vi "main.vi"() -> ()   [LabVIEW 2019]
uses:
  Controls/States.ctl
  Controls/Data.ctl
panel:
  in  "Exit":bool
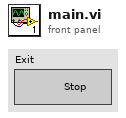
[diagram p1: front panel]
types:
  T1 = typedef "Data.ctl" = cluster{"Data":dbl[], "Info":string}
  T2 = typedef "States.ctl" = enum16{"Inizialize", "Wait for event", "Calculate", "Clear", "Exit"}
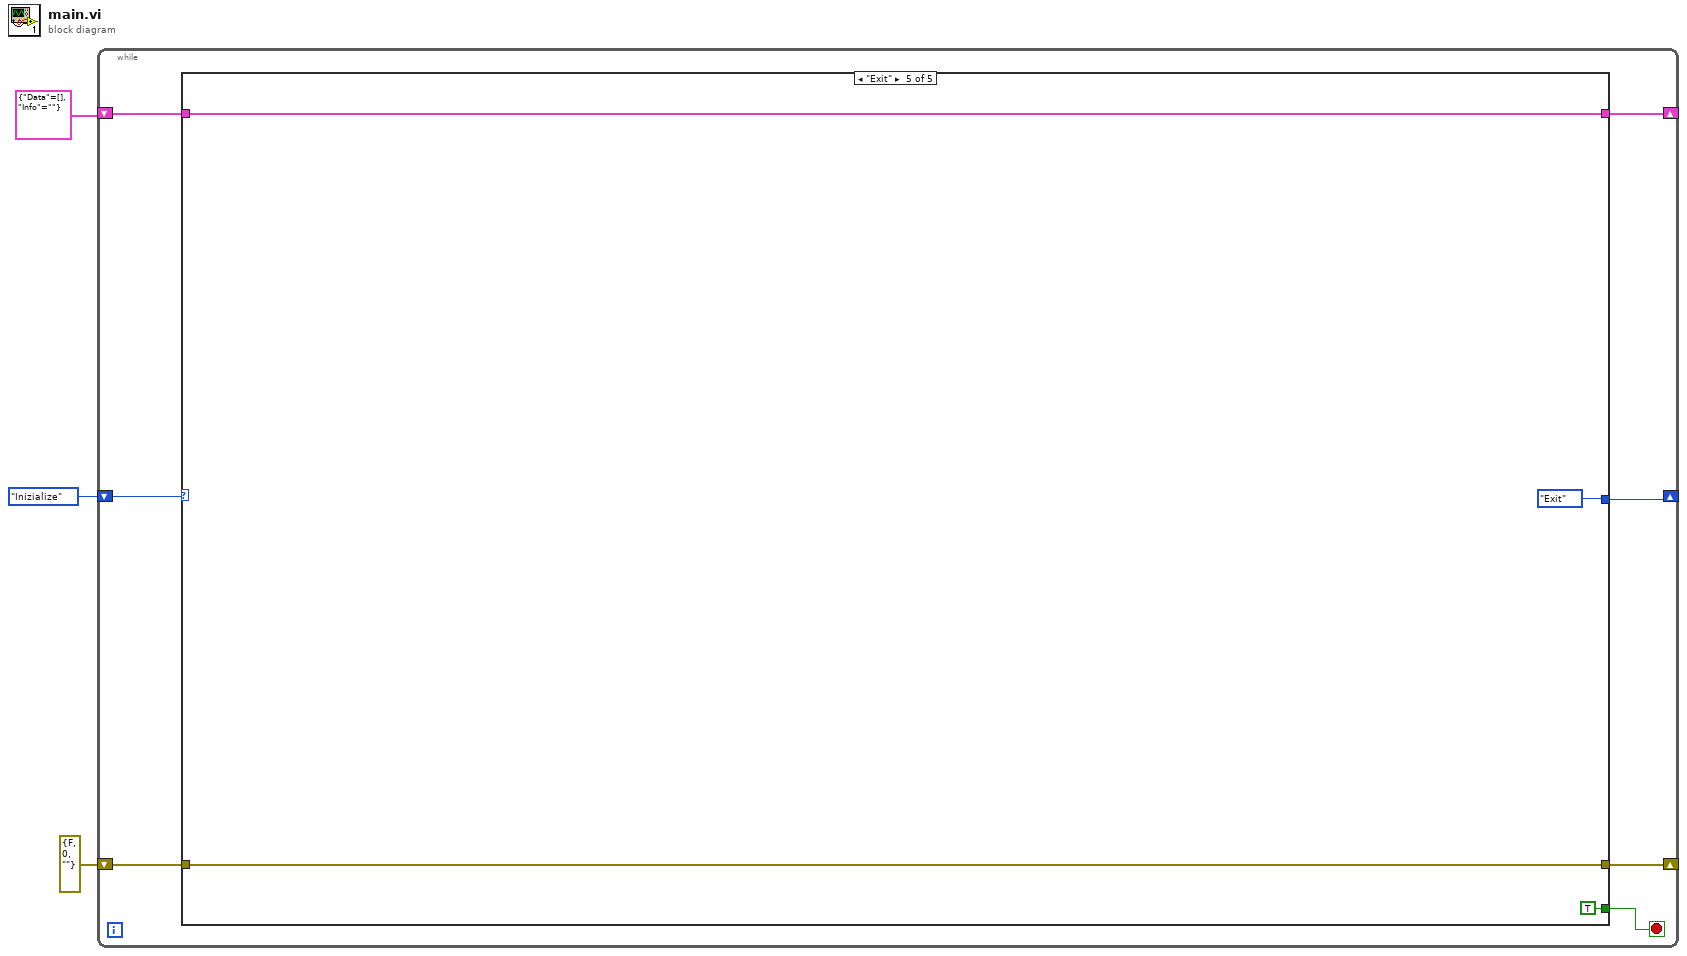
[diagram p0: block diagram]
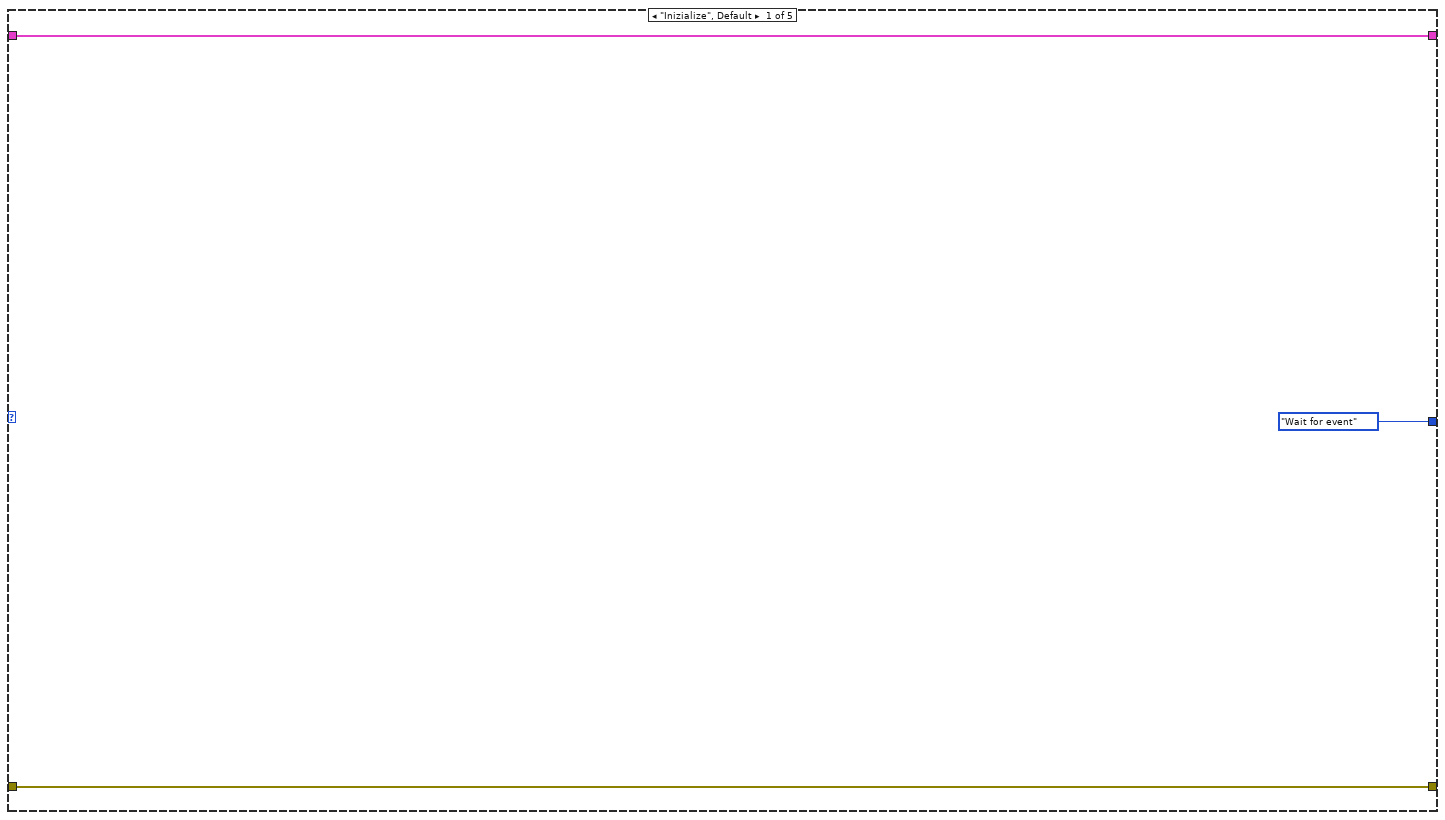
[diagram p2: hidden frame]
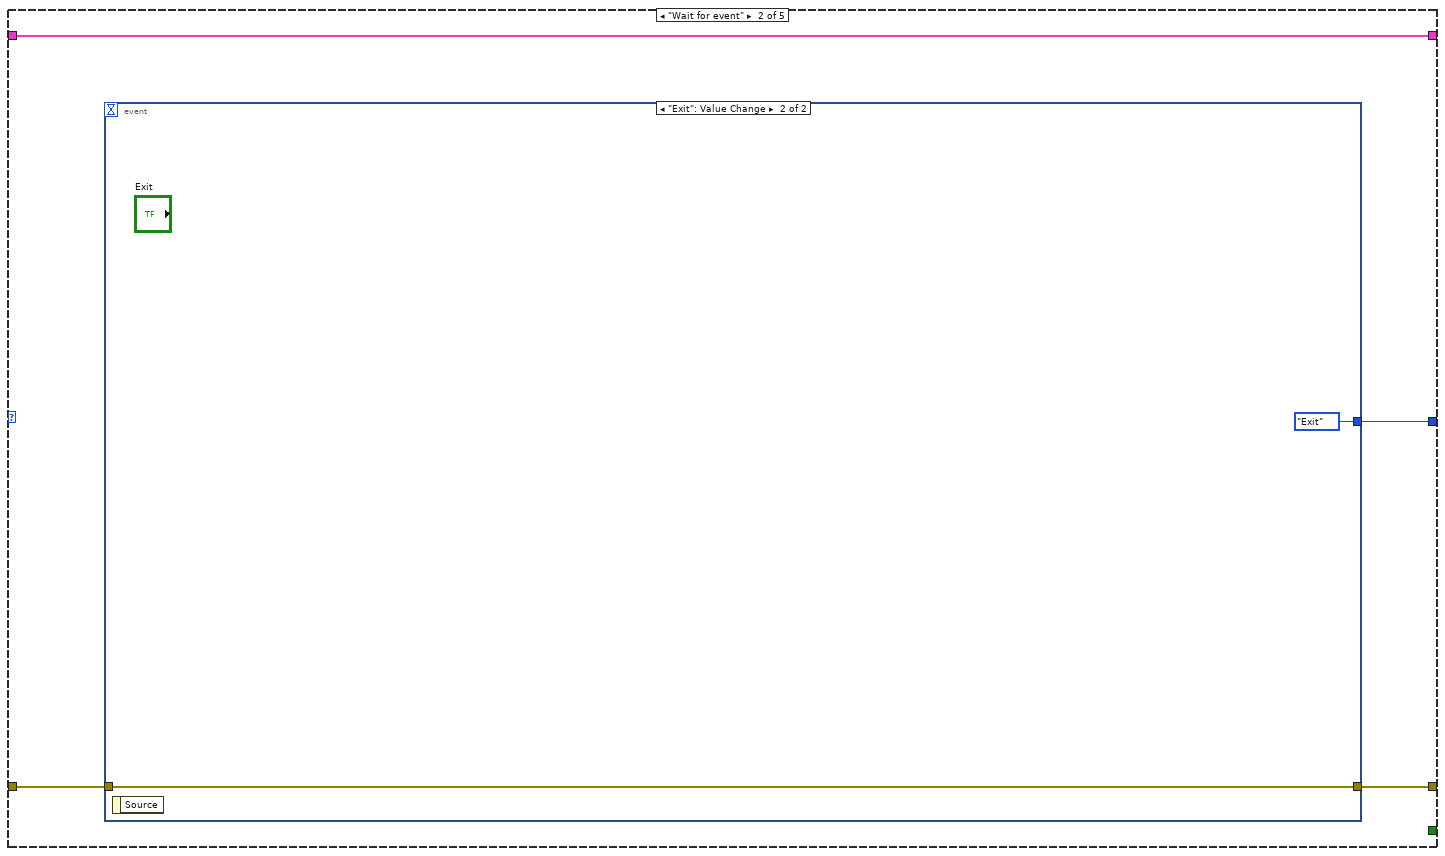
[diagram p3: hidden frame]
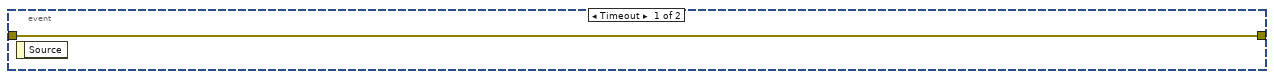
[diagram p4: hidden frame]
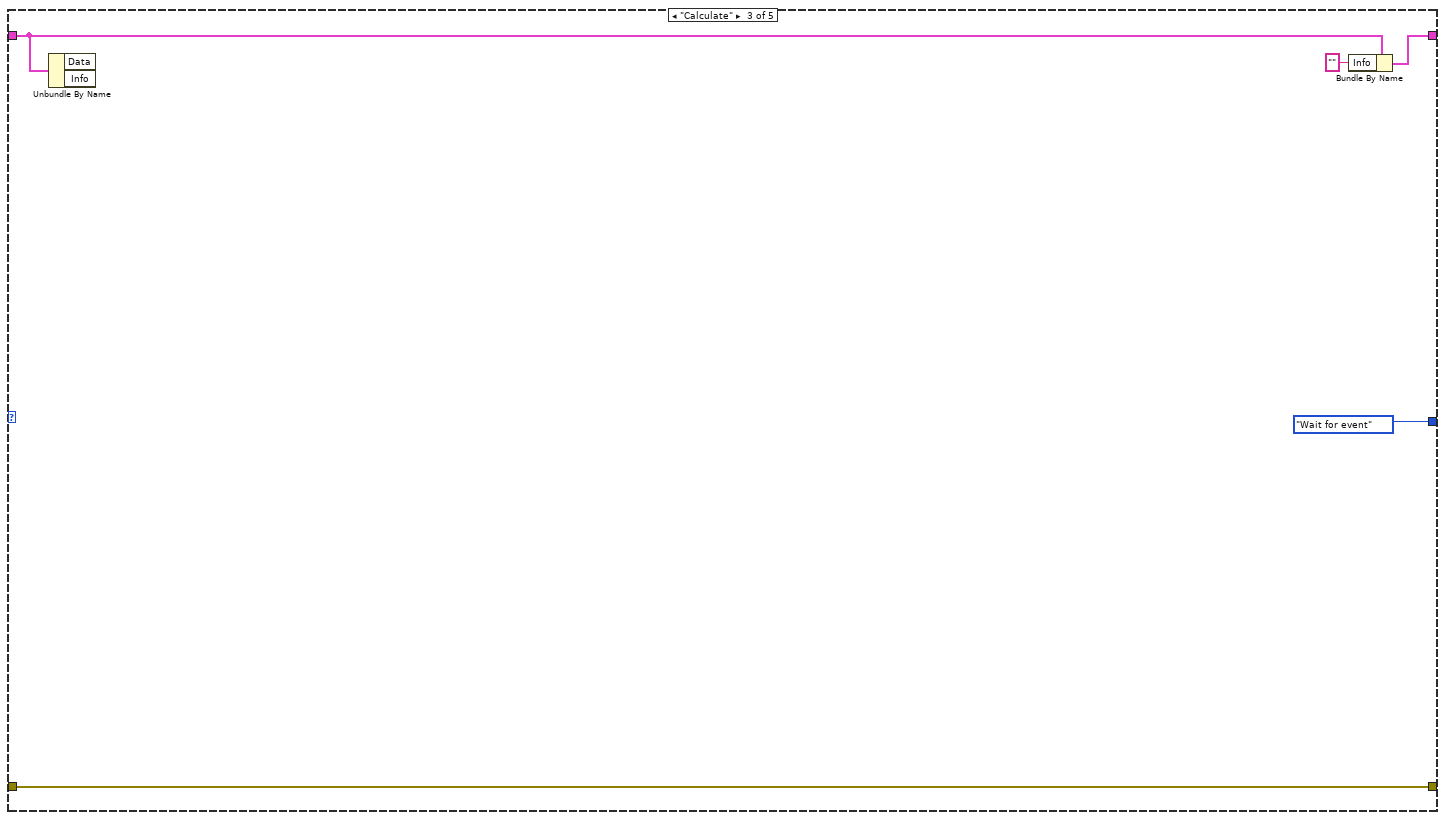
[diagram p5: hidden frame]
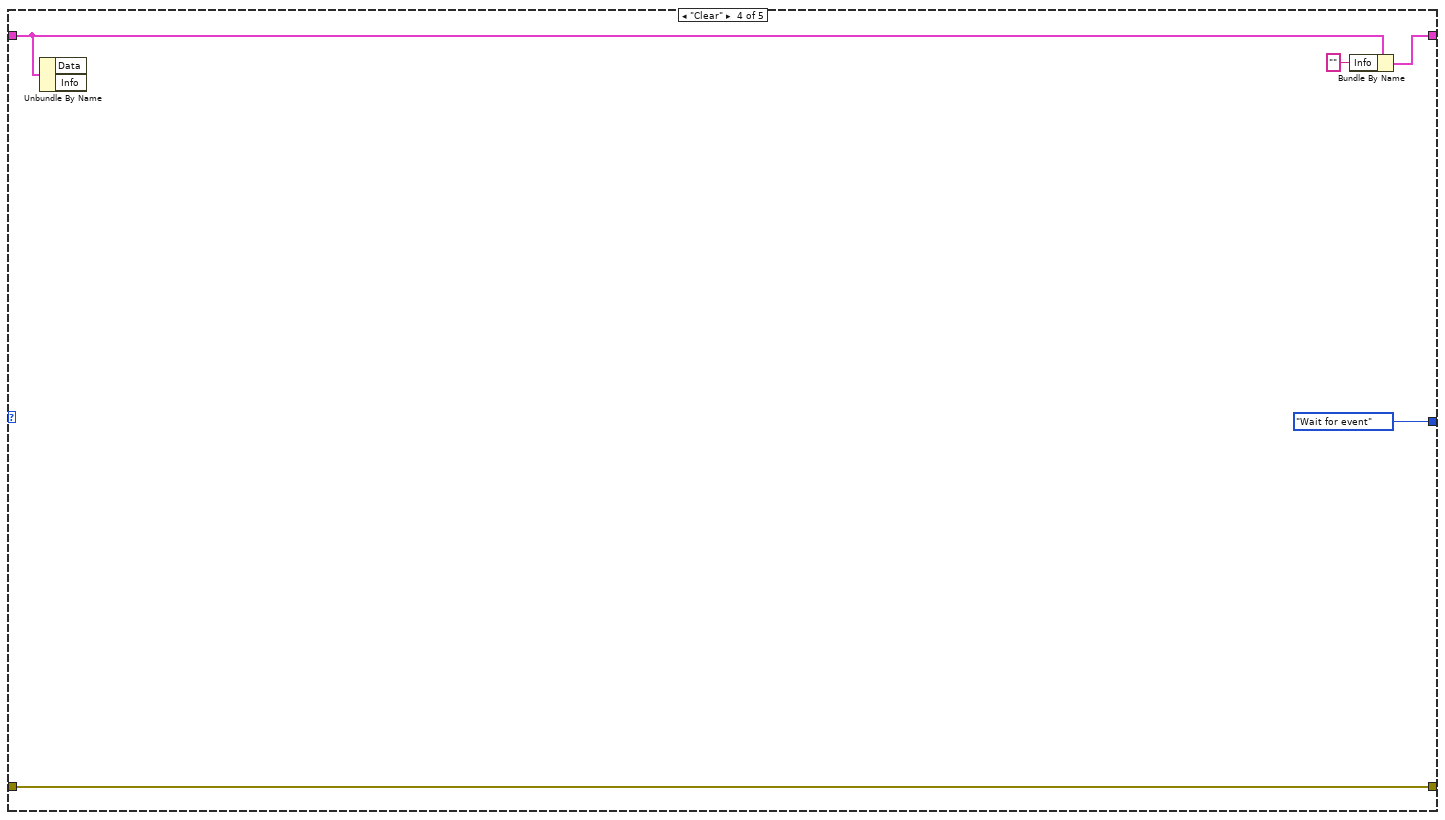
[diagram p6: hidden frame]
diagram:
  n1 = while {
    shift-right: [w9] -> _
    shift-left: States."Inizialize" ("Enum") -> [w10]
    shift-right: [w8] -> _
    shift-left: T1 {"Data"=[], "Info"=""} ("Data") -> [w7]
    shift-right: [w4] -> _
    shift-left: errorcluster {"status"=FALSE, "code"=0, "source"=""} ("error in (no error)") -> [w5]
    stop <- w6 stop-if-true
    n2 = case shown="\"Exit\"" w10 {
      tunnel: [States."Wait for event" ("Enum") w17 States."Wait for event" ("Enum") States."Wait for event" ("Enum") States."Exit" ("Enum")] -> w9
      tunnel: [w13 w16 w23 w28 w34] -> w8
      tunnel: w7 -> [w13 w16 w24 w29 w34]
      tunnel: [_ _ _ _ TRUE] -> w6
      tunnel: w5 -> [w12 w15 w25 w30 w31]
      tunnel: [w12 w14 w25 w30 w31] -> w4
      frame "Inizialize", Default {
      }
      frame "Wait for event" {
        n3 = event shown="[1] \"Exit\": Value Change" {
          selector: _ -> [_ _]
          dyn-events: _ -> [_ _]
          timeout: _ -> [_ _]
          tunnel: [_ States."Exit" ("Enum")] -> w17
          tunnel: [w18 w19] -> w14
          tunnel: w15 -> [w18 w19]
          event Timeout {
            n4 = event-data() -> ()  [unwired: 1 in, 1 out]
          }
          event "Exit": Value Change {
            n5 = event-data() -> ()  [unwired: 1 in, 1 out]
          }
        }
      }
      frame "Calculate" {
        n6 = Unbundle By Name(w24) -> ()  [unwired: 2 out]
        n7 = Bundle By Name(cluster=w24, "Info"="") -> (w23:T1)
      }
      frame "Clear" {
        n8 = Unbundle By Name(w29) -> ()  [unwired: 2 out]
        n9 = Bundle By Name(cluster=w29, "Info"="") -> (w28:T1)
      }
      frame "Exit" {
      }
    }
  }
